vi "CodigoLabView.vi"() -> ()   [LabVIEW 2025]
uses:
  <vilib>/Instr/_visa.llb/VISA Configure Serial Port (Instr).vi
panel:
  in  "Relé N°2":bool
  in  "Relé N°1":bool
  out "Serial Settings:Number of Bytes at Serial Port":u32
  out "error out 2":errorcluster
  out "Enviando":string
  out "error out":errorcluster
  out "Meter":dbl(knob) scale=0.0..5.0 scale format="%#_6f"
  out "Numeric":dbl
  out "String":string
  in  "VISA resource name":refnum<visa-resource-name>
  in  "stop":bool
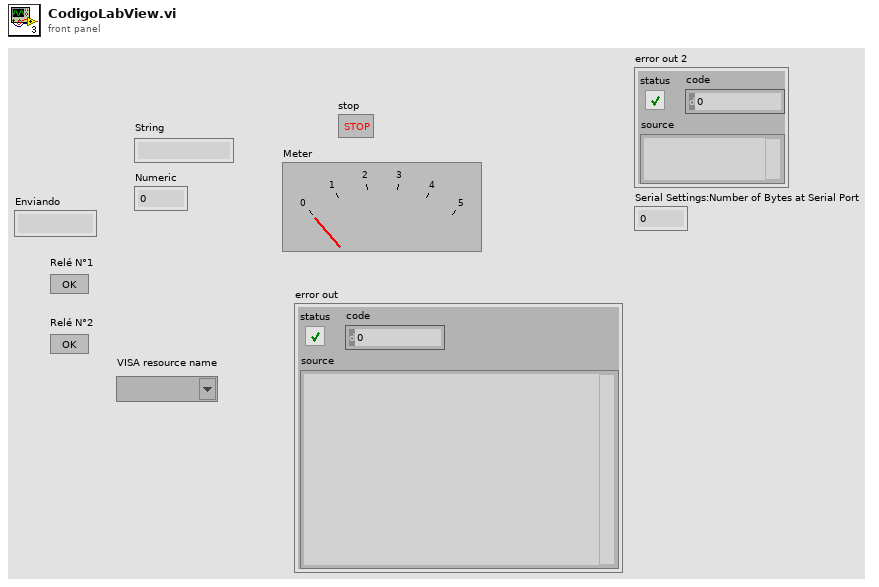
[diagram p1: front panel]
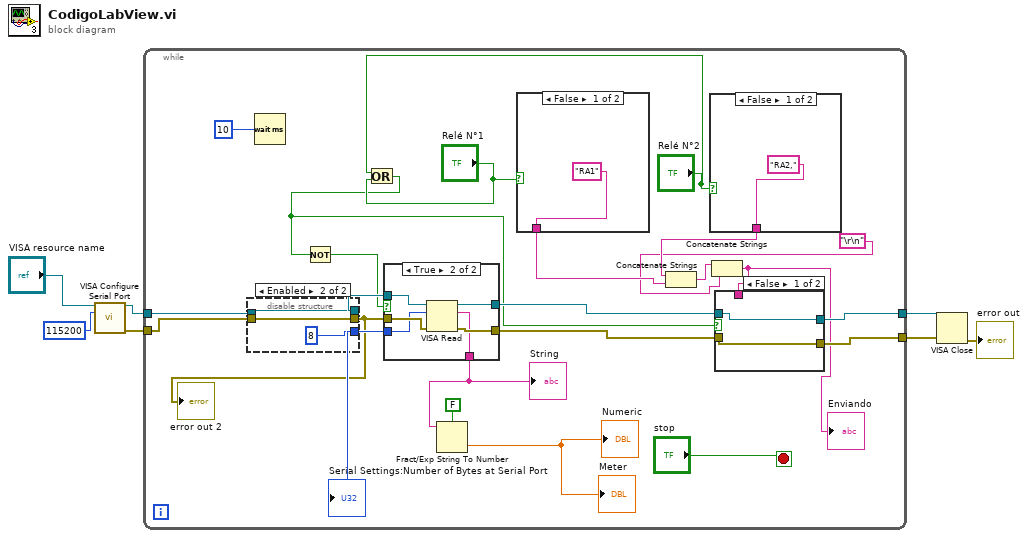
[diagram p0: block diagram]
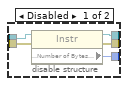
[diagram p2: hidden frame]
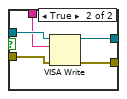
[diagram p4: hidden frame]
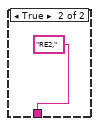
[diagram p5: hidden frame]
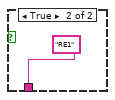
[diagram p6: hidden frame]
diagram:
  n1 = call-poly "VISA Configure Serial Port"("VISA resource name"="VISA resource name", "baud rate (9600)"=u32 115200) -> ("VISA resource name out"=w7:refnum<visa-resource-name>, "error out"=w1:errorcluster)  [unwired: 12 in]
  n2 = while {
    tunnel: w7 -> [w29]
    tunnel: [w23] -> w6
    tunnel: w1 -> [w28]
    tunnel: [w22] -> w5
    stop <- "stop" stop-if-true
    n3 = disable-structure shown="Enabled" {
      disable-tunnel: w29 -> [w35 w38]
      disable-tunnel: w28 -> [w34 w37]
      disable-tunnel: [w33 w38] -> w17
      disable-tunnel: [w32 u32 8 ("Bytes at Port")] -> w16
      disable-tunnel: [w31 w37] -> w14
      frame Disabled {
        n4 = property class="Instr"(reference=w35, error in=w34) -> (reference out=w33:refnum<visa-resource-name>, error out=w31:errorcluster, "Serial Settings:Number of Bytes at Serial Port"=w32:u32)
      }
      frame Enabled {
      }
    }
    "error out 2" <- w14
    "Serial Settings:Number of Bytes at Serial Port" <- w16
    n5 = Wait (ms)(milliseconds to wait=u32 10) -> ()  [unwired: 1 out]
    n6 = Or(x="Relé N°2", y="Relé N°1") -> (x .or. y?=w10:bool)
    n7 = Not(x=w10) -> (.not. x?=w11:bool)
    n8 = case shown="True" w11 {
      tunnel: [w40 w46] -> w19
      tunnel: [w39 w45] -> w18
      tunnel: w14 -> [w39 w44]
      tunnel: w17 -> [w40 w43]
      tunnel: w16 -> [_ w42]
      tunnel: [_ w41] -> w15
      frame False {
      }
      frame True {
        n9 = VISA Read(VISA resource name=w43, byte count=w42, error in (no error)=w44) -> (VISA resource name out=w46:refnum<visa-resource-name>, read buffer=w41:string, error out=w45:errorcluster)  [unwired: 1 out]
      }
    }
    "String" <- w15
    n10 = Fract/Exp String To Number(use system decimal point (T)=FALSE, string=w15) -> (number=→"Numeric" →"Meter":dbl)  [unwired: 2 in, 1 out]
    n11 = case shown="False" "Relé N°1" {
      tunnel: ["RA1" "RE1"] -> w25
      frame False {
      }
      frame True {
      }
    }
    n12 = case shown="False" "Relé N°2" {
      tunnel: ["RA2," "RE2,"] -> w24
      frame False {
      }
      frame True {
      }
    }
    n13 = Concatenate Strings(w24, w25) -> (w20:string)
    n14 = Concatenate Strings(w20, "\r\n") -> (w21:string)
    "Enviando" <- w21
    n15 = case shown="False" w10 {
      tunnel: [w48 w53] -> w23
      tunnel: [w47 w52] -> w22
      tunnel: w19 -> [w48 w51]
      tunnel: w18 -> [w47 w50]
      tunnel: w21 -> [_ w49]
      frame False {
      }
      frame True {
        n16 = VISA Write(VISA resource name=w51, write buffer=w49, error in (no error)=w50) -> (VISA resource name out=w53:refnum<visa-resource-name>, error out=w52:errorcluster)  [unwired: 1 out]
      }
    }
  }
  n17 = VISA Close(VISA resource name=w6, error in (no error)=w5) -> (error out=→"error out":errorcluster)
